vi "Grab images from pco.edge or pco.pixelfly CL debug.vi"() -> ()   [LabVIEW 2015]
doc: "A short program to demonstrate the fundamentals of control and image acquision with the pco.camera series. The program records a sequence of images, with \"live\" updating, until the \"StopRecording\" button is pressed. Use ctrl-H for more help on the individual controls and indicators.\n\nCopyright 2004, 2010 The Cooke Corporation."
panel:
  out "Count":i32
  out "PageSize":u16
  out "RamSize":u32
  out "ActSeg":u16=1 min=1 max=4 step=1
  out "x-y 4":dbl format="%#_4f"
  out "x-y 3":dbl format="%#_4f"
  out "x-y 2":dbl format="%#_4f"
  out "Numeric":i32
  out "x-y":dbl format="%#_4f"
  out "StorageMode":bool
  out "RecorderSubMode":bool
  out "AcquireEnableInUse":bool
  out "Transfer Parameters":T1
  out "ImageTiming":T2
  out "FrameRate":dbl format="%#.3f"
  out "Waveform Chart":dbl(graph)
  out "cam_fps":dbl=20.079713544692744 caption="FPS" format="%.1g"
  out "bClose":bool
  in  "Quit":bool
  out "BufNr1":i16
  out "BufNr0":i16
  in  "bUseBuffer1":bool
  in  "bUseBuffer0":bool
  in  "ROIX1":u16=1 min=1
  in  "ROIY1":u16=1 min=1
  in  "ROIY0":u16=1 min=1
  in  "ROIX0":u16=1 min=1
  out "Bits/pixel":u16
  in  "Record":bool
  in  "DelayTimeBase":u16(ring)=2 items=["nanoseconds", "microseconds", "milliseconds"]
  in  "ExposureTimeBase":u16(ring)=2 items=["nanoseconds", "microseconds", "milliseconds"]
  in  "Exposure":u32=10
  in  "Delay":u32
  in  "Rate":i32(ring) items=["95333333", "286000000"]
  out "Image":u16[][](graph)
  in  "TriggerMode":u16(ring) items=["Auto", "Software", "External sequence start ", "External exposure control"]
  # "A short program to demonstrate the fundamentals of control and image acquision with the pco.camera series. The program records a sequence of images, with \"live\" updating, until the \"StopRecording\" button is pressed.  Use ctrl-H for more help on the individual controls and indicators."
  # "pco.labview"
  # "1) Setup camera:"
  # "2) Record  images:"
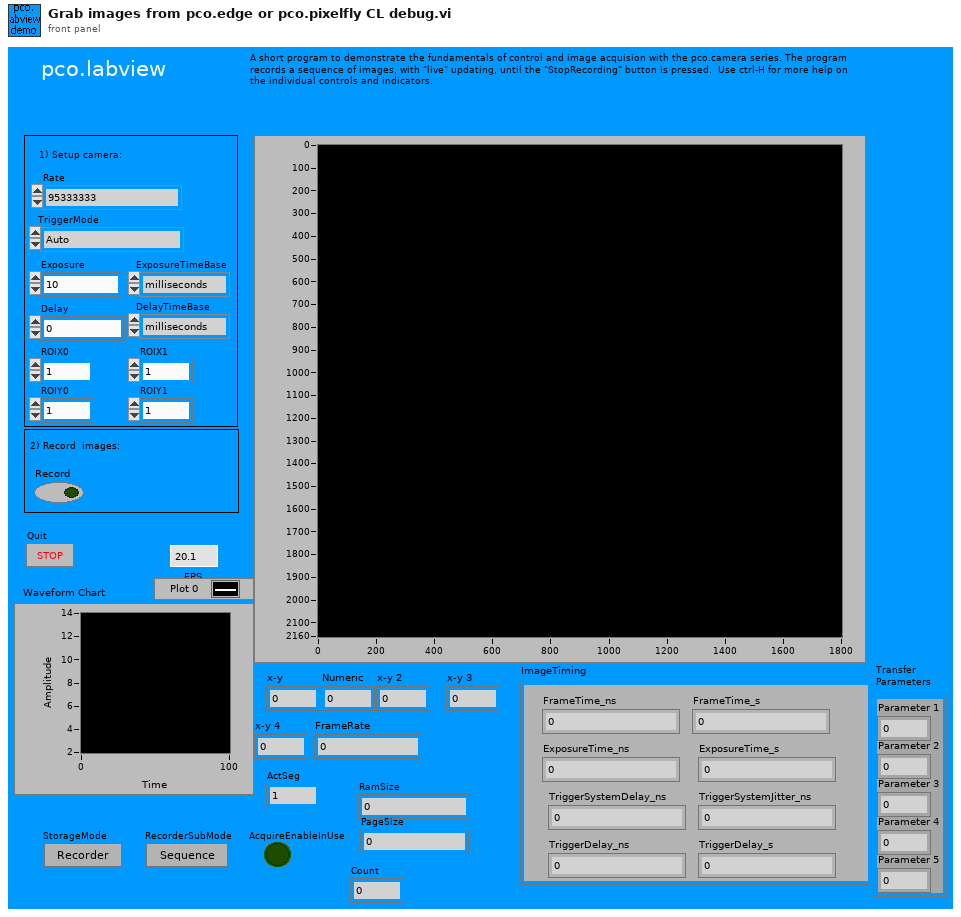
[diagram p1: front panel]
types:
  T1 = cluster{"Parameter 1":u32, "Parameter 2":u32, "Parameter 3":u32, "Parameter 4":u32, "Parameter 5":u32}
  T2 = cluster{"FrameTime_ns":u32, "FrameTime_s":u32, "ExposureTime_ns":u32, "ExposureTime_s":u32, "TriggerSystemDelay_ns":u32, "TriggerSystemJitter_ns":u32, "TriggerDelay_ns":u32, "TriggerDelay_s":u32}
  T3 = cluster{"SSize":u16, "CamType":u16, "CamsSubType":u16, "SerialNumber":u32, "HWVersion":u32, "FWVersion ":u32, "InterfaceType":u16, "HardwareVersions":cluster{"Board":u16, cluster{"string":string, "BatchNumber":u16, "MinorRevision":u8, "MajorRevision":u8, "Variant":u16}[]}, "FirmwareVersions":cluster{"DeviceNum":u16, cluster{"string":string, "MinorRevision":u8, "MajorRevision":u8, "Variant":u16}[]}}
  T4 = cluster{"Size":u16, "SensorTypeDESC":u16, "SensorSubtypeDESC":u16, "MaxHorizontalResStdDESC":u16, "MaxVerticalResStdDESC":u16, "MaxHorizontalResExtDESC":u16, "MaxVerticalResExtDESC":u16, "DynResDESC":u16, "MaxBinHorzDESC":u16, "BinHorzStepDESC":bool, "MaxBinVertDESC":u16, "BinVertStepDESC":bool, "ROIHorzStepDESC":u16, "ROIVertStepDESC":u16, "NumADCDESC":u16, "IRDESC":bool, "MinDelayDESC":u32, "MaxDelayDESC":u32, "MinDelayStepDESC":u32, "MinExpoDESC":u32, "MaxExpoDESC":u32, "MinExpoStepDESC":u32, "MinDelayIRDESC":u32, "MaxDelayIRDESC":u32, "MinExpoIRDESC":u32, "MaxExpoIRDESC":u32, "TimeTableDESC":bool, "DoubleImageDESC":bool, "MinCoolSetDESC":i16, "MaxCoolSetDESC":i16, "MDefaultCoolSetDESC":i16, "PowerDownModeDESC":bool, "OffsetRegDESC":bool, "ColorPattern":cluster{"UpperLeftColor":u8, "UpperRightColor":u8, "LowerLeftColor":u8, "LowerRightColor":u8}, "PatternTypeDESC":bool, "PixelRates":u32[], "CoversionFactors":u16[], "Reserved":u32[], "GeneralCapabilities":u32, "GeneralCapabilities 2":u32, "Min Size Hor":u16, "Min Size Vert":u16, "Ext Synch Freq":u32[], "Cooling Setpoints":i16[], "Soft ROI Hor Step":u16, "Soft ROI Vert Step":u16}
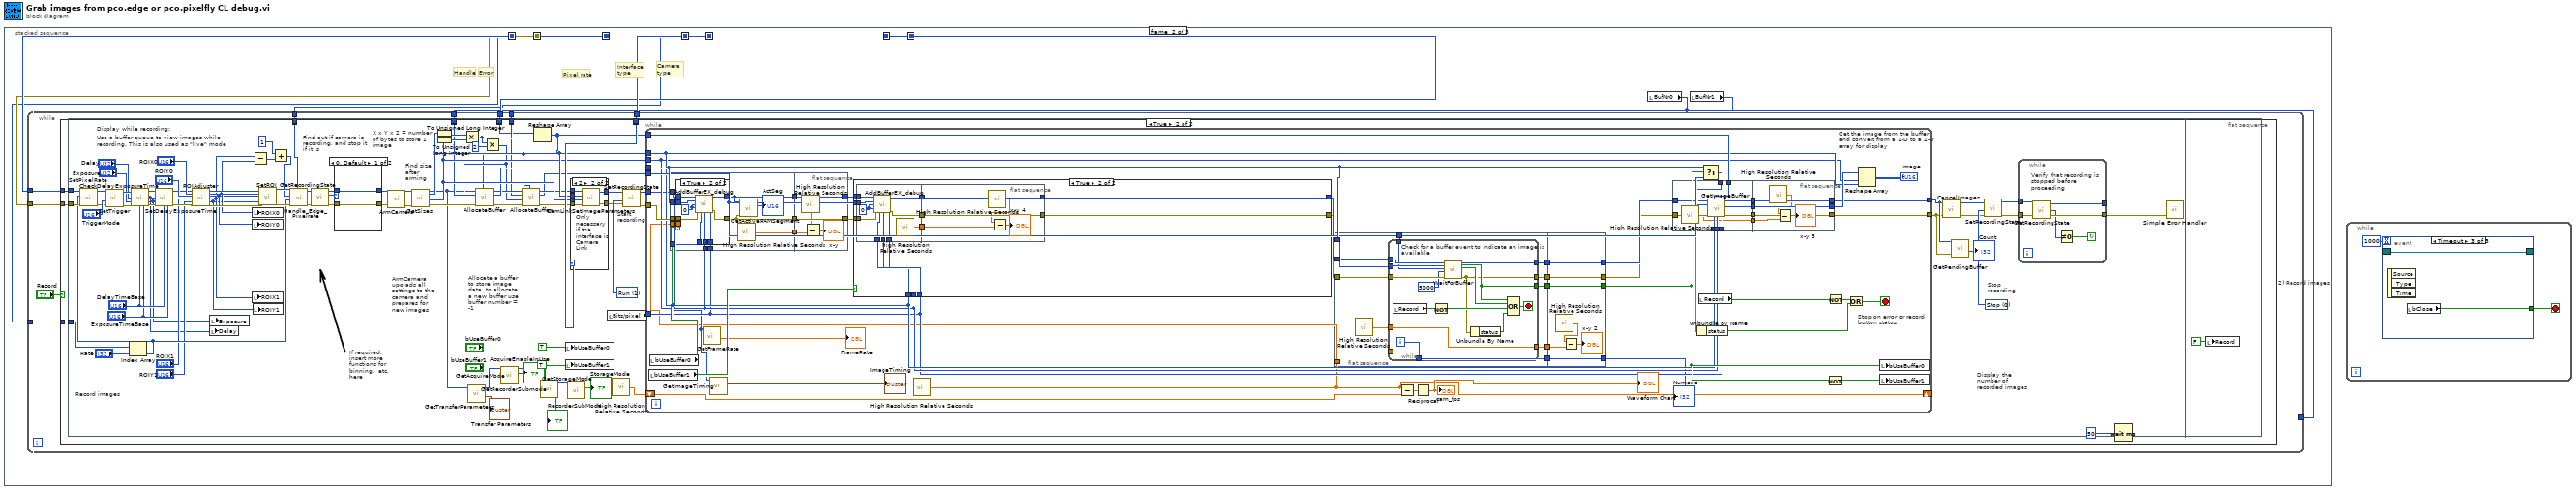
[diagram p0: block diagram]
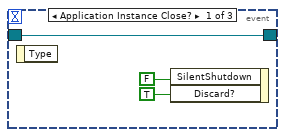
[diagram p2: hidden frame]
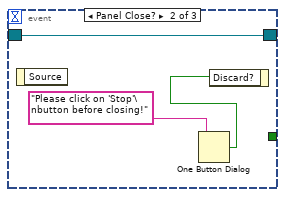
[diagram p3: hidden frame]
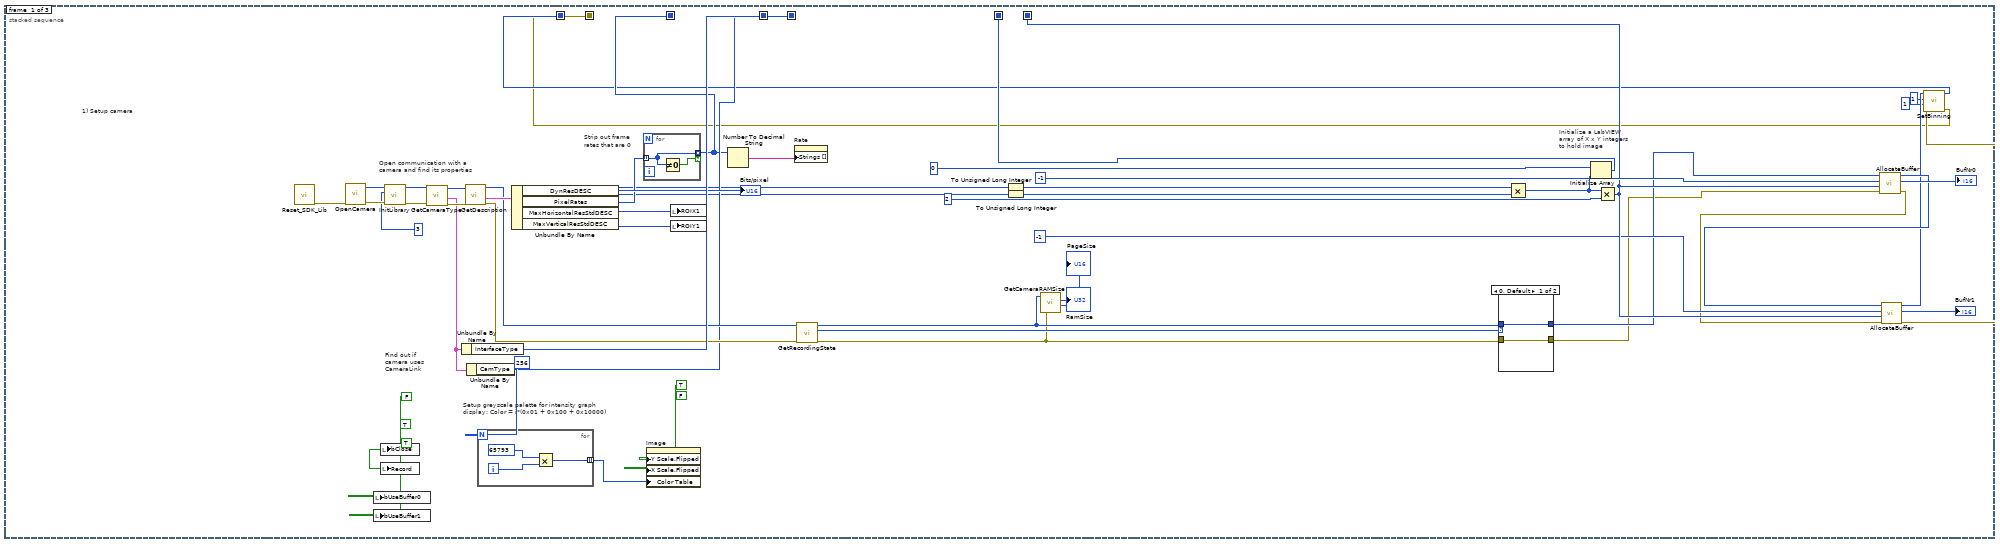
[diagram p4: hidden frame]
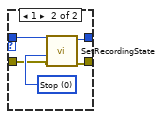
[diagram p5: hidden frame]
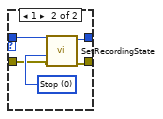
[diagram p10: hidden frame]
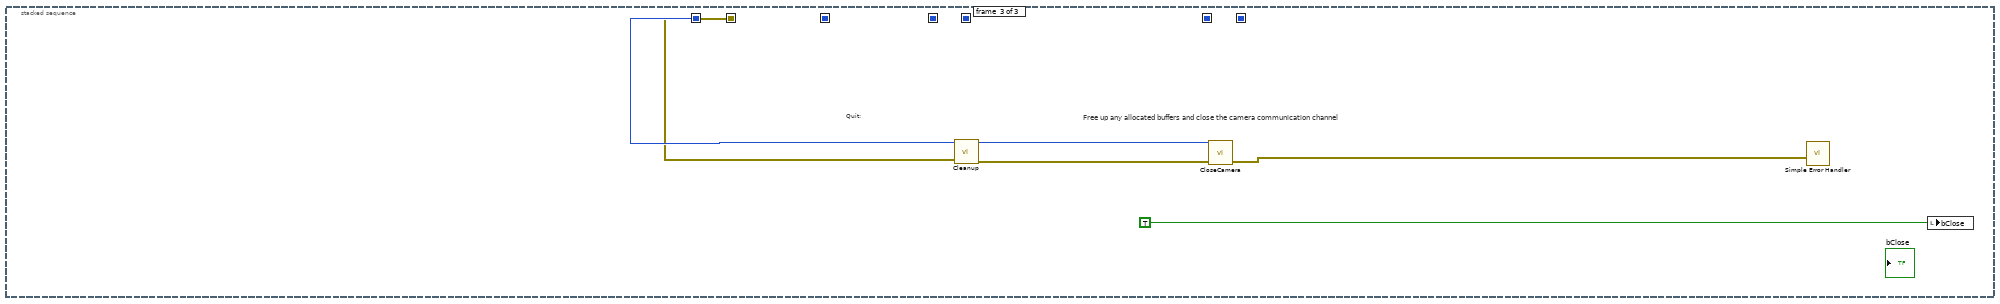
[diagram p11: hidden frame]
diagram:
  # "Camera type"
  # "Interface type"
  # "Error"
  # "Handle"
  # "Pixel rate"
  n1 = stacked-sequence {
    seq-local: [w47 _ _] -> [_ w70 _]
    seq-local: [w37 _ _] -> [_ _ _]
    seq-local: [w11 _ _] -> [_ w73 w358]
    seq-local: [w9 _ _] -> [_ w72 w357]
    seq-local: [w42 _ _] -> [_ w71 _]
    seq-local: [w13 _ _] -> [_ w67 _]
    seq-local: [w15 _ _] -> [_ w66 _]
    frame #0 {
      w31 = FALSE ("stop")
      # "Strip out frame rates that are 0"
      # "1) Setup camera"
      # "Find out if camera uses CameraLink"
      # "Setup greyscale palette for intensity graph display: Color = i*(0x01 + 0x100 + 0x10000)"
      # "Initialize a LabVIEW array of X x Y integers to hold image"
      # "Open communication with a camera and find its properties"
      n2 = call "Reset_SDK_Lib.vi"() -> ("ErrorOut"=w17:errorcluster)  [unwired: 11 in]
      n3 = call "OpenCamera.vi"("ErrorIn"=w17) -> ("ErrorOut"=w28:errorcluster, "Handle out"=w29:u64)  [unwired: 3 in, 2 out]
      n4 = local write "bUseBuffer0"(TRUE) -> ()
      n5 = local write "bUseBuffer1"(TRUE) -> ()
      n6 = local write "bClose"(w31) -> ()
      n7 = local write "Record"(w31) -> ()
      n8 = call "InitLibrary.vi"("error in (no error)"=w28, "InterfaceType"=u32 3, "ph"=w29) -> ("error out"=w27:errorcluster, "hout"=w26:u64)  [unwired: 7 in]
      n9 = call "GetCameraType.vi"("ph"=w26, "error in (no error)"=w27) -> ("hout"=w44:u64, "CameraType"=w16:T3, "error out"=w43:errorcluster)  [unwired: 1 in, 1 out]
      n10 = Unbundle By Name(w16) -> ("InterfaceType"=w42:u16)
      n11 = call "GetDescription.vi"("ErrorIn"=w43, "ph"=w44) -> ("ErrorOut"=w23:errorcluster, "Description"=w46:T4, "hout"=w22:u64)  [unwired: 2 in, 1 out]
      n12 = Unbundle By Name(w16) -> ("CamType"=w15:u16)
      n13 = for {
        N: 256 -> [_]
        tunnel: [w63] -> w50 mode=indexing
        i -> [w64]
        n14 = Multiply(x=65793, y=w64) -> (x*y=w63:i32)
      }
      n15 = Unbundle By Name(w46) -> ("DynResDESC"=→"Bits/pixel":u16, "PixelRates"=w14:u32[], "MaxHorizontalResStdDESC"=w7:u16, "MaxVerticalResStdDESC"=w8:u16)
      n16 = for {
        tunnel: w14 -> [w54] mode=indexing
        tunnel: [w54] -> w13 mode=indexing if=w55
        n17 = Not Equal To 0?(x=w54) -> (x != 0?=w55:bool)
      }
      n18 = property on="Image" class="IntGraph (strict)"("Y Scale.Flipped"=TRUE, "X Scale.Flipped"=FALSE, "Color Table"=w50) -> ()  [unwired: 2 in, 2 out]
      n19 = local write "ROIX1"(w7) -> ()
      n20 = local write "ROIY1"(w8) -> ()
      n21 = Number To Decimal String(number=w13) -> (decimal integer string=w30:string[])  [unwired: 1 in]
      n22 = property on="Rate" class="Ring (strict)"("Strings []"=w30) -> ()  [unwired: 2 in, 2 out]
      n23 = call "GetRecordingState.vi"("ErrorIn"=w23, "ph"=w22) -> ("ErrorOut"=w3:errorcluster, "Error"=w18:i32, "hout"=w4:u64)  [unwired: 2 in, 1 out]
      n24 = To Unsigned Long Integer(number=w7) -> (unsigned 32bit integer=w39:u32)
      n25 = To Unsigned Long Integer(number=w8) -> (unsigned 32bit integer=w38:u32)
      n26 = call "GetCameraRAMSize.vi"("ph"=w4, "error in (no error)"=w3) -> ("RamSize"=→"RamSize":u32, "PageSize"=→"PageSize":u16)  [unwired: 1 in, 3 out]
      n27 = case shown="0, Default" w18 {
        tunnel: w4 -> [w57 w61]
        tunnel: w3 -> [w56 w60]
        tunnel: [w57 w59] -> w21
        tunnel: [w56 w58] -> w19
        frame 0, Default {
        }
        frame 1 {
          w62 = u16 0 items=["Stop", "Run"] ("RecordingState")
          n28 = call "SetRecordingState.vi"("ErrorIn"=w60, "RecordingState"=w62, "ph"=w61) -> ("ErrorOut"=w58:errorcluster, "hout"=w59:u64)  [unwired: 2 in, 1 out]
        }
      }
      n29 = Multiply(x=w39, y=w38) -> (x*y=w48:u32)
      n30 = Initialize Array(u16 0 ("Element Data"), w48) -> (w47:u16[])
      n31 = Multiply(x=w48, y=u32 2) -> (x*y=w37:u32)
      n32 = call "AllocateBuffer.vi"("error in (no error)"=w19, "Size"=w37, "BufNr"=i16 -1, "ph"=w21) -> ("error out"=w24:errorcluster, "BufNrOut"=→"BufNr0":i16, "hout"=w20:u64)  [unwired: 2 in, 3 out]
      n33 = call "AllocateBuffer.vi"("error in (no error)"=w24, "Size"=w37, "BufNr"=i16 -1, "ph"=w20) -> ("error out"=w10:errorcluster, "BufNrOut"=→"BufNr1":i16, "hout"=w12:u64)  [unwired: 2 in, 3 out]
      n34 = call "SetBinning.vi"("error in (no error)"=w10, "BinVert"=u16 1, "BinHorz"=u16 1, "ph"=w12) -> ("error out"=w9:errorcluster, "hout"=w11:u64)  [unwired: 3 in, 1 out]
    }
    frame #1 {
      n35 = local read "BufNr0"() -> (w69:i16)
      n36 = local read "BufNr1"() -> (w68:i16)
      n37 = while {
        tunnel: w69 -> [_]
        tunnel: w69 -> [w79]
        tunnel: w70 -> [w81]
        tunnel: w71 -> [w82]
        tunnel: w72 -> [w80]
        tunnel: w73 -> [w77]
        tunnel: w68 -> [w78]
        tunnel: w67 -> [w75]
        tunnel: w66 -> [w74]
        stop <- "Quit" stop-if-true
        n38 = case "2) Record images" shown="True" "Record" {
          tunnel: w77 -> [_ w92]
          tunnel: w80 -> [_ w91]
          tunnel: w82 -> [_ w90]
          tunnel: w81 -> [_ w89]
          tunnel: w79 -> [_ w88]
          tunnel: w78 -> [_ w87]
          tunnel: w75 -> [_ w86]
          tunnel: w74 -> [_ w85]
          frame False {
          }
          frame True {
            n39 = flat-sequence {
              tunnel: w92 -> [w167]
              tunnel: w91 -> [w166]
              tunnel: w90 -> [w164]
              tunnel: w89 -> [w94]
              tunnel: w88 -> [w155]
              tunnel: w87 -> [w149]
              tunnel: w86 -> [w138]
              tunnel: w85 -> [w129]
              frame #0 {
                w179 = u16 1 items=["Stop", "Run"] ("RecordingState")
                w182 = u16 0 items=["Stop", "Run"] ("RecordingState")
                # "Display the number of recorded images"
                # "Record images"
                # "Start recording"
                # "Allocate a buffer to store image data. to allocate a new buffer use buffer number = -1"
                # "Find size after arming"
                # "ArmCamera upolads all settings to the camera and prepares for new images"
                # "Find out if camera is recording, and stop it if it is"
                # "If required, insert more functions for binning.  etc. here"
                # "X x Y x 2 = number of bytes to store 1 image"
                # "Stop recording"
                # "Use a buffer queue to view images while recording. This is also used as \"live\" mode"
                # "Display while recording:"
                n40 = Index Array(array=w138, index="Rate") -> (element=w133:u32)
                n41 = call "SetPixelRate.vi"("error in (no error)"=w166, "PixelRate"=w133, "ph"=w167) -> ("error out"=w140:errorcluster, "hout"=w141:u64)  [unwired: 2 in, 1 out]
                n42 = call "SetTrigger.vi"("error in (no error)"=w140, "TriggerMode"="TriggerMode", "ph"=w141) -> ("error out"=w118:errorcluster, "hout"=w120:u64)  [unwired: 2 in, 1 out]
                n43 = call "CheckDelayExposureTime.vi"("ph"=w120, "Delay"="Delay", "Exposure"="Exposure", "error in (no error)"=w118, "DelayTimeBase"="DelayTimeBase", "ExposureTimeBase"="ExposureTimeBase") -> ("hout"=w119:u64, "Delay Out"=w112:u32, "Exposure Out"=w111:u32, "error out"=w113:errorcluster)  [unwired: 4 in, 2 out]
                n44 = call "SetDelayExposureTime.vi"("ph"=w119, "Delay"=w112, "Exposure"=w111, "error in (no error)"=w113, "DelayTimeBase"="DelayTimeBase", "ExposureTimeBase"="ExposureTimeBase") -> ("hout"=w122:u64, "error out"=w128:errorcluster)  [unwired: 7 in, 1 out]
                n45 = call "ROIAdjuster.vi"("HandleIn"=w122, "ROIXmin"="ROIX0", "ROIYmin"="ROIY0", "ROIXmax"="ROIX1", "ROIYmax"="ROIY1", "ErrorIn"=w128) -> ("hout"=w121:u64, "ROIX0Mod"=w101:u16, "ROIY0Mod"=w100:u16, "ROIX1Mod"=w99:u16, "ROIY1Mod"=w98:u16, "ErrorOut"=w127:errorcluster)  [unwired: 7 in, 1 out]
                n46 = local write "Delay"(w112) -> ()
                n47 = local write "Exposure"(w111) -> ()
                n48 = Subtract(x=w99, y=w101) -> (x-y=w132:u16)
                n49 = local write "ROIX0"(w101) -> ()
                n50 = local write "ROIY0"(w100) -> ()
                n51 = local write "ROIX1"(w99) -> ()
                n52 = local write "ROIY1"(w98) -> ()
                n53 = call "SetROI.vi"("ph"=w121, "ROIX0"=w101, "ROIY0"=w100, "ROIX1"=w99, "ROIY1"=w98, "error in (no error)"=w127) -> ("hout"=w134:u64, "error out"=w135:errorcluster)  [unwired: 12 in]
                n54 = Add(x=1, y=w132) -> (x+y=w130:i32)
                n55 = call "Handle_Edge_Pixelrate.vi"("Cameratype"=w129, "error in (no error)"=w135, "PixelRate"=w133, "X-Resolution"=w130, "ph"=w134) -> ("error out"=w136:errorcluster, "hout"=w137:u64)  [unwired: 5 in]
                n56 = call "GetRecordingState.vi"("ErrorIn"=w136, "ph"=w137) -> ("ErrorOut"=w176:errorcluster, "RecordingState"=w178:u16, "hout"=w177:u64)  [unwired: 2 in, 1 out]
                n57 = case shown="0, Default" w178 {
                  tunnel: w177 -> [w350 w354]
                  tunnel: w176 -> [w349 w353]
                  tunnel: [w350 w352] -> w175
                  tunnel: [w349 w351] -> w174
                  frame 0, Default {
                  }
                  frame 1 {
                    w355 = u16 0 items=["Stop", "Run"] ("RecordingState")
                    n58 = call "SetRecordingState.vi"("ErrorIn"=w353, "RecordingState"=w355, "ph"=w354) -> ("ErrorOut"=w351:errorcluster, "hout"=w352:u64)  [unwired: 2 in, 1 out]
                  }
                }
                n59 = call "ArmCamera.vi"("error in (no error)"=w174, "ph"=w175) -> ("error out"=w172:errorcluster, "hout"=w173:u64)  [unwired: 1 in, 1 out]
                n60 = call "GetSizes.vi"("ph"=w173, "ErrorIn"=w172) -> ("hout"=w109:u64, "XResAct"=w162:u16, "YResAct"=w161:u16, "ErrorOut"=w171:errorcluster)  [unwired: 11 in, 3 out]
                n61 = To Unsigned Long Integer(number=w162) -> (unsigned 32bit integer=w156:u32)
                n62 = To Unsigned Long Integer(number=w161) -> (unsigned 32bit integer=w157:u32)
                n63 = Multiply(x=w156, y=w157) -> (x*y=w158:u32)
                n64 = call "GetTransferParameters.vi"("ph"=w109) -> ("Transfer Parameters"=→"Transfer Parameters":T1, "hout"=w108:u64)  [unwired: 3 in, 2 out]
                n65 = Multiply(x=w158, y=u32 2) -> (x*y=w150:u32)
                n66 = call "GetAcquireMode.vi"("ph"=w108) -> ("AcquireEnableInUse"=→"AcquireEnableInUse":bool, "hout"=w107:u64)  [unwired: 3 in, 2 out]
                n67 = Reshape Array(w94, w158) -> (w93:u16[])
                n68 = call "AllocateBuffer.vi"("BufIn"=w93, "error in (no error)"=w171, "Size"=w150, "BufNr"=w155, "ph"=w109) -> ("error out"=w154:errorcluster, "BufNrOut"=w159:i16, "hout"=w152:u64)  [unwired: 1 in, 3 out]
                n69 = call "AllocateBuffer.vi"("BufIn"=w93, "error in (no error)"=w154, "Size"=w150, "BufNr"=w149, "ph"=w152) -> ("error out"=w153:errorcluster, "BufNrOut"=w148:i16, "hout"=w151:u64)  [unwired: 1 in, 3 out]
                n70 = call "GetRecorderSubmode.vi"("ph"=w107) -> ("RecorderSubMode"=→"RecorderSubMode":bool, "hout"=w106:u64)  [unwired: 3 in, 2 out]
                n71 = local write "bUseBuffer0"(TRUE) -> ()
                n72 = local write "bUseBuffer1"(TRUE) -> ()
                n73 = call "GetStorageMode.vi"("ph"=w106) -> ("StorageMode"=→"StorageMode":bool)  [unwired: 3 in, 3 out]
                n74 = case shown="2" w164 {
                  tunnel: w153 -> [w341 w348]
                  tunnel: [w341 w347] -> w169
                  tunnel: w151 -> [w342 w346]
                  tunnel: [w342 w345] -> w168
                  tunnel: w161 -> [_ w344]
                  tunnel: w162 -> [_ w343]
                  frame 0, Default {
                  }
                  frame 2 {
                    # "Only necessary if the interface is Camera Link"
                    n75 = call "CamLinkSetImageParameters.vi"("error in (no error)"=w348, "YRes"=w344, "XRes"=w343, "ph"=w346) -> ("error out"=w347:errorcluster, "hout"=w345:u64)  [unwired: 1 out]
                  }
                }
                n76 = local read "Bits/pixel"() -> (w143:u16)
                n77 = call <vilib>:"High Resolution Relative Seconds.vi"() -> ("relative seconds"=w110:dbl)
                n78 = call "SetRecordingState.vi"("ErrorIn"=w169, "RecordingState"=w179, "ph"=w168) -> ("ErrorOut"=w165:errorcluster, "hout"=w163:u64)  [unwired: 2 in, 1 out]
                n79 = while {
                  tunnel: w159 -> [w215]
                  tunnel: w93 -> [w224]
                  tunnel: w163 -> [w198]
                  tunnel: w161 -> [w204]
                  tunnel: w162 -> [w205]
                  tunnel: w165 -> [w222]
                  tunnel: [w226] -> w97
                  tunnel: [w227] -> w96
                  tunnel: w148 -> [w214]
                  tunnel: w143 -> [w203]
                  shift-right: [w195] -> _
                  shift-left: w110 -> [w201]
                  stop <- w206 stop-if-true
                  # "Stop on error or record button status"
                  # "Get the image from the buffer and convert from a 1-D to a 2-D array for display"
                  n80 = local read "bUseBuffer1"() -> (w219:bool)
                  n81 = local read "bUseBuffer0"() -> (w220:bool)
                  n82 = flat-sequence {
                    tunnel: w222 -> [w240]
                    tunnel: w220 -> [w239]
                    tunnel: w215 -> [w238]
                    tunnel: w205 -> [w237]
                    tunnel: w204 -> [w236]
                    tunnel: w203 -> [w235]
                    tunnel: w198 -> [w234]
                    tunnel: w195 -> [w233]
                    tunnel: [w231] -> w185
                    tunnel: [w230] -> w184
                    tunnel: [w232] -> w183
                    tunnel: [w255] -> w221
                    tunnel: [w256] -> w223
                    tunnel: w185 -> [w256]
                    tunnel: w184 -> [w255]
                    tunnel: w183 -> [w254]
                    frame #0 {
                      n83 = case shown="True" w239 {
                        tunnel: [w242 w251] -> w230
                        tunnel: [w241 w250] -> w231
                        tunnel: w238 -> [_ w249]
                        tunnel: w234 -> [w241 w248]
                        tunnel: w235 -> [_ w246]
                        tunnel: w237 -> [_ w245]
                        tunnel: w236 -> [_ w244]
                        tunnel: w240 -> [w242 w243]
                        tunnel: w233 -> [_ _]
                        frame False {
                        }
                        frame True {
                          w247 = i16 0
                          n84 = call "AddBufferEX_debug.vi"("ph"=w248, "BuffNr"=w249, "1stImage"=w247, "LastImage"=w247, "error in (no error)"=w243, "XRes"=w245, "YRes"=w244, "BitPerPixel"=w246) -> ("hout"=w250:u64, "error out"=w251:errorcluster)  [unwired: 5 in, 1 out]
                        }
                      }
                      n85 = call <vilib>:"High Resolution Relative Seconds.vi"() -> ("relative seconds"=w232:dbl)
                      n86 = call "GetActiveRAMSegment.vi"("error in (no error)"=w230, "ph"=w231) -> ("ActSeg"=→"ActSeg":u16)  [unwired: 2 in, 3 out]
                    }
                    frame #1 {
                      n87 = call <vilib>:"High Resolution Relative Seconds.vi"() -> ("relative seconds"=w253:dbl)
                      n88 = Subtract(x=w253, y=w254) -> (x-y=→"x-y":dbl)
                    }
                  }
                  n89 = call "GetFrameRate.vi"("ph"=w198) -> ("FrameRate"=→"FrameRate":dbl)  [unwired: 3 in, 5 out]
                  n90 = call "GetImageTiming.vi"("ph"=w198) -> ("ImageTiming"=→"ImageTiming":T2)  [unwired: 4 in, 3 out]
                  n91 = case shown="True" w219 {
                    tunnel: [w307 w319] -> w212
                    tunnel: [w308 w318] -> w213
                    tunnel: w214 -> [_ w317]
                    tunnel: w223 -> [w308 w316]
                    tunnel: w203 -> [_ w315]
                    tunnel: w205 -> [_ w314]
                    tunnel: w204 -> [_ w313]
                    tunnel: w221 -> [w307 w312]
                    frame False {
                    }
                    frame True {
                      n92 = flat-sequence {
                        tunnel: w317 -> [w327]
                        tunnel: w316 -> [w326]
                        tunnel: w315 -> [w324]
                        tunnel: w314 -> [w323]
                        tunnel: w313 -> [w322]
                        tunnel: w312 -> [w321]
                        tunnel: [w329] -> w311
                        tunnel: [w328] -> w310
                        tunnel: [w320] -> w309
                        tunnel: [w333] -> w318
                        tunnel: [w334] -> w319
                        tunnel: w311 -> [w334]
                        tunnel: w310 -> [w333]
                        tunnel: w309 -> [w332]
                        frame #0 {
                          w325 = i16 0
                          n93 = call "AddBufferEX_debug.vi"("ph"=w326, "BuffNr"=w327, "1stImage"=w325, "LastImage"=w325, "error in (no error)"=w321, "XRes"=w323, "YRes"=w322, "BitPerPixel"=w324) -> ("hout"=w328:u64, "error out"=w329:errorcluster)  [unwired: 5 in, 1 out]
                          n94 = call <vilib>:"High Resolution Relative Seconds.vi"() -> ("relative seconds"=w320:dbl)
                        }
                        frame #1 {
                          n95 = call <vilib>:"High Resolution Relative Seconds.vi"() -> ("relative seconds"=w331:dbl)
                          n96 = Subtract(x=w331, y=w332) -> (x-y=→"x-y 4":dbl)
                        }
                      }
                    }
                  }
                  n97 = call <vilib>:"High Resolution Relative Seconds.vi"() -> ("relative seconds"=w195:dbl)
                  n98 = flat-sequence {
                    tunnel: w215 -> [w284]
                    tunnel: w214 -> [w283]
                    tunnel: w213 -> [w282]
                    tunnel: w212 -> [w281]
                    tunnel: w195 -> [w276]
                    tunnel: [w280] -> w194
                    tunnel: [w279] -> w193
                    tunnel: [w278] -> w192
                    tunnel: [w277] -> w191
                    tunnel: [w275] -> w190
                    tunnel: [w303] -> w196
                    tunnel: [w304] -> w209
                    tunnel: [w305] -> w210
                    tunnel: [w306] -> w211
                    tunnel: w194 -> [w306]
                    tunnel: w193 -> [w305]
                    tunnel: w192 -> [w304]
                    tunnel: w191 -> [w303]
                    tunnel: w190 -> [w301]
                    frame #0 {
                      n99 = call <vilib>:"High Resolution Relative Seconds.vi"() -> ("relative seconds"=w274:dbl)
                      n100 = while {
                        tunnel: w284 -> [w294]
                        tunnel: w283 -> [w293]
                        tunnel: w282 -> [w296]
                        tunnel: w281 -> [w295]
                        tunnel: [w292] -> w280
                        tunnel: [w288] -> w278
                        tunnel: [w291] -> w279
                        tunnel: [w286] -> w277
                        tunnel: w276 -> [_]
                        tunnel: [w285] -> w275
                        tunnel: w274 -> [w285]
                        i -> [w286]
                        stop <- w297 stop-if-true
                        # "Check for a buffer event to indicate an image is available"
                        n101 = local read "Record"() -> (w299:bool)
                        n102 = Not(x=w299) -> (.not. x?=w298:bool)
                        n103 = call "WaitForBuffer.vi"("ph"=w296, "sBufNr"=w294, "sBufNr 2"=w293, "timeout"=5000, "error in (no error)"=w295) -> ("hout"=w292:u64, "Buffer_Ready"=w291:bool, "Buffer_Ready 2"=w290:bool, "error out"=w288:errorcluster)  [unwired: 10 in, 1 out]
                        n104 = Unbundle By Name(w288) -> ("status"=w287:bool)
                        n105 = Compound Arithmetic op=OR(w291, w290, w298, w287) -> (w297:bool)
                      }
                    }
                    frame #1 {
                      n106 = call <vilib>:"High Resolution Relative Seconds.vi"() -> ("relative seconds"=w302:dbl)
                      n107 = Subtract(x=w302, y=w301) -> (x-y=→"x-y 2":dbl)
                    }
                  }
                  n108 = Subtract(x=w195, y=w201) -> (x-y=w202:dbl)
                  n109 = Reciprocal(x=w202) -> (1/x=→"cam_fps" →"Waveform Chart":dbl)
                  n110 = flat-sequence {
                    tunnel: w224 -> [w264]
                    tunnel: w218 -> [w263]
                    tunnel: w211 -> [w262]
                    tunnel: w209 -> [w261]
                    tunnel: w205 -> [w260]
                    tunnel: w204 -> [w259]
                    tunnel: w203 -> [w258]
                    tunnel: [w267] -> w189
                    tunnel: [w266] -> w188
                    tunnel: [w265] -> w187
                    tunnel: [w257] -> w186
                    tunnel: [w271] -> w226
                    tunnel: [w272] -> w227
                    tunnel: [w273] -> w228
                    tunnel: w189 -> [w273]
                    tunnel: w188 -> [w272]
                    tunnel: w187 -> [w271]
                    tunnel: w186 -> [w268]
                    frame #0 {
                      n111 = call <vilib>:"High Resolution Relative Seconds.vi"() -> ("relative seconds"=w257:dbl)
                      n112 = call "GetImageBuffer.vi"("ph"=w262, "BuffIn"=w264, "BuffNr"=w263, "error in (no error)"=w261, "xRes"=w260, "yRes"=w259, "Bitresolution"=w258) -> ("hout"=w265:u64, "BuffOut"=w267:u16[], "error out"=w266:errorcluster)  [unwired: 5 in, 1 out]
                    }
                    frame #1 {
                      n113 = call <vilib>:"High Resolution Relative Seconds.vi"() -> ("relative seconds"=w269:dbl)
                      n114 = Subtract(x=w269, y=w268) -> (x-y=→"x-y 3":dbl)
                    }
                  }
                  n115 = Unbundle By Name(w209) -> ("status"=w207:bool)
                  n116 = local read "Record"() -> (w225:bool)
                  n117 = Select(t=w215, s=w210, f=w214) -> (s? t:f=w218:i16)
                  n118 = Not(x=w210) -> (.not. x?=w217:bool)
                  n119 = Not(x=w225) -> (.not. x?=w208:bool)
                  n120 = Or(x=w208, y=w207) -> (x .or. y?=w206:bool)
                  n121 = Reshape Array(w228, w204, w205) -> (→"Image":u16[][])
                  n122 = local write "bUseBuffer0"(w210) -> ()
                  n123 = local write "bUseBuffer1"(w217) -> ()
                  "Numeric" <- w196
                }
                n124 = call "CancelImages.vi"("error in (no error)"=w96, "ph"=w97) -> ("error out"=w145:errorcluster, "hout"=w144:u64)  [unwired: 1 in, 1 out]
                n125 = call "GetPendingBuffer.vi"("ph"=w97, "error in (no error)"=w96) -> ("Count"=→"Count":i32)  [unwired: 1 in, 3 out]
                n126 = call "SetRecordingState.vi"("ErrorIn"=w145, "RecordingState"=w182, "ph"=w144) -> ("ErrorOut"=w180:errorcluster, "hout"=w181:u64)  [unwired: 2 in, 1 out]
                n127 = while {
                  tunnel: [w338] -> w142
                  tunnel: w180 -> [w339]
                  tunnel: w181 -> [w340]
                  tunnel: [w335] -> _
                  stop <- w336 continue-if-true
                  # "Verify that recording is stopped before proceeding"
                  n128 = call "GetRecordingState.vi"("ErrorIn"=w339, "ph"=w340) -> ("ErrorOut"=w338:errorcluster, "RecordingState"=w337:u16, "hout"=w335:u64)  [unwired: 2 in, 1 out]
                  n129 = Not Equal To 0?(x=w337) -> (x != 0?=w336:bool)
                }
                n130 = call <vilib>:"Simple Error Handler.vi"("error in (no error)"=w142) -> ()  [unwired: 4 in, 5 out]
              }
              frame #1 {
                n131 = local write "Record"(FALSE ("Record")) -> ()
              }
            }
          }
        }
        n132 = Wait (ms)(milliseconds to wait=u32 50) -> ()  [unwired: 1 out]
      }
    }
    frame #2 {
      # "Free up any allocated buffers and close the camera communication channel"
      # "Quit:"
      n133 = call "Cleanup.vi"("error in (no error)"=w357, "ph"=w358) -> ("error out"=w359:errorcluster, "hout"=w360:u64)  [unwired: 8 in]
      n134 = call "CloseCamera.vi"("ErrorIn"=w359, "Handle in"=w360) -> ("ErrorOut"=w362:errorcluster)  [unwired: 1 in, 2 out]
      n135 = call <vilib>:"Simple Error Handler.vi"("error in (no error)"=w362) -> ()  [unwired: 4 in, 5 out]
      n136 = local write "bClose"(TRUE) -> ()
    }
  }
  n137 = while {
    stop <- w363 stop-if-true
    n138 = event shown="[2] Timeout" {
      selector: _ -> [w365 w370 w372]
      dyn-events: [w365 w370 w372] -> _
      timeout: 1000 -> [_ _ _]
      tunnel: [_ _ w371] -> w363
      event Application Instance Close? {
        n139 = event-data() -> ()  [unwired: 1 in, 1 out]
        n140 = event-data("SilentShutdown"=FALSE, "Discard?"=TRUE) -> ()  [unwired: 1 in, 1 out]
      }
      event Panel Close? {
        n141 = event-data() -> ()  [unwired: 1 in, 1 out]
        n142 = One Button Dialog(message="Please click on 'Stop'\nbutton before closing!") -> (true=w368:bool)  [unwired: 1 in]
        n143 = event-data("Discard?"=w368) -> ()  [unwired: 1 in, 1 out]
      }
      event Timeout {
        n144 = event-data() -> ()  [unwired: 1 in, 3 out]
        n145 = local read "bClose"() -> (w371:bool)
      }
    }
  }
